vi "ReadBestRecord.vi"(7 "IndexColumn":i32=3, 8 "ErrorInput":errorcluster, 11 "FilepathInput":path=path "C:/Users/jinbeom/Desktop/data.txt") -> (0 "ErrorOutput":errorcluster, 2 "Data":string[](array[string]), 3 "FilepathOutput":path)   [LabVIEW 2020]
uses:
  <vilib>/Utility/file.llb/Read Delimited Spreadsheet (string).vi
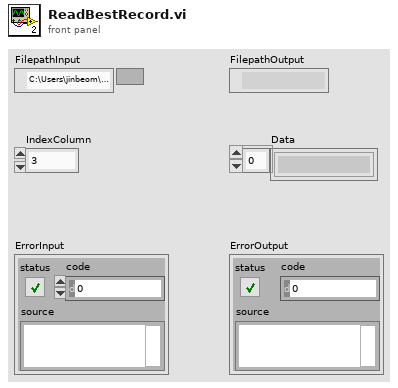
[diagram p1: front panel]
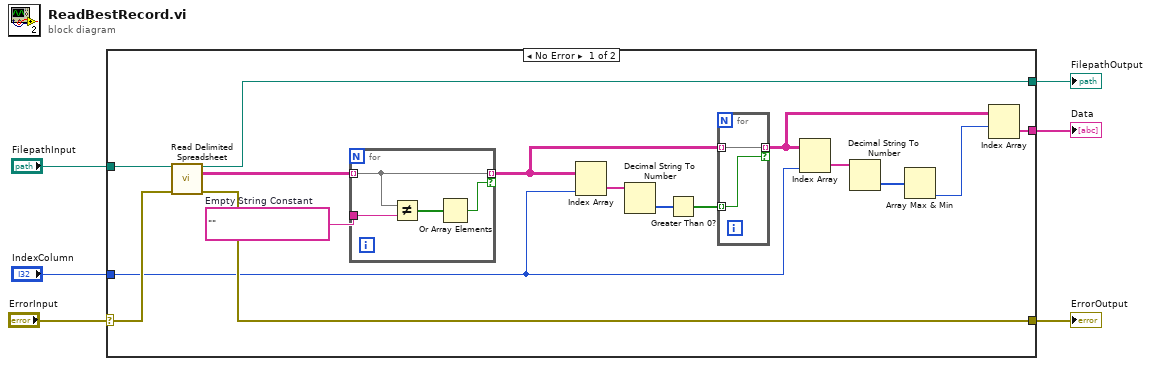
[diagram p0: block diagram]
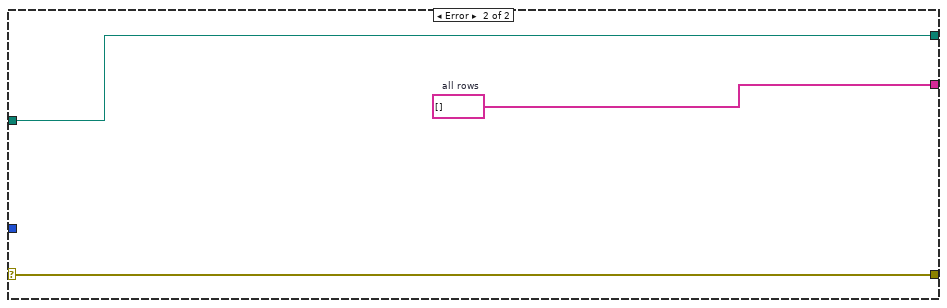
[diagram p2: hidden frame]
diagram:
  n1 = case shown="No Error" "ErrorInput" {
    selector: "ErrorInput" -> [w15 w31]
    tunnel: "FilepathInput" -> [w22 w30]
    tunnel: "IndexColumn" -> [w10 _]
    tunnel: [w20 w29] -> w4
    tunnel: [w18 w30] -> w3
    tunnel: [w16 w31] -> w1
    frame No Error {
      w14 = ""  # Empty String Constant
      n2 = call-poly <vilib>:"Read Delimited Spreadsheet.vi"("file path (dialog if empty)"=w22, "error in (no error)"=w15) -> ("new file path (Not A Path if cancelled)"=w18:path, "all rows"=w17:string[][], "error out"=w16:errorcluster)  [unwired: 8 in, 3 out]
      n3 = for {
        tunnel: w17 -> [w28] mode=indexing
        tunnel: [w28] -> w11 mode=indexing if=w26
        tunnel: w14 -> [w25]
        n4 = Not Equal?(x=w28, y=w25) -> (x != y?=w27:bool[])
        n5 = Or Array Elements(Boolean array=w27) -> (logical OR=w26:bool)
      }
      n6 = Index Array "Index Array"(array=w11, index (col)=w10) -> (element=w19:string[])  [unwired: 1 in]
      n7 = Decimal String To Number(string=w19) -> (number=w13:i32[])  [unwired: 2 in, 1 out]
      n8 = Greater Than 0?(x=w13) -> (x > 0?=w12:bool[])
      n9 = for {
        tunnel: w12 -> [w23] mode=indexing
        tunnel: w11 -> [w24] mode=indexing
        tunnel: [w24] -> w7 mode=indexing if=w23
      }
      n10 = Index Array "Index Array"(array=w7, index (col)=w10) -> (element=w9:string[])  [unwired: 1 in]
      n11 = Decimal String To Number(string=w9) -> (number=w8:i32[])  [unwired: 2 in, 1 out]
      n12 = Array Max & Min(array=w8) -> (min index (indices)=w21:i32)  [unwired: 3 out]
      n13 = Index Array "Index Array"(array=w7, index (row)=w21) -> (element=w20:string[])  [unwired: 1 in]
    }
    frame Error {
      w29 = string[] []  # all rows
    }
  }
  "Data" <- w4
  "FilepathOutput" <- w3
  "ErrorOutput" <- w1
